vi "Set Message Type.vi"(6 "EF20 Message type":T1 items=["Update", "Graph", "Status", "Parameter", "Acknowledge"], 8 "error in":errorcluster, 11 "EF20 in":refnum<class "EF20.lvclass">) -> (0 "error out":errorcluster, 3 "EF20 out":refnum<class "EF20.lvclass">)   [LabVIEW 2018, in "EF20.lvlib" / "EF20.lvclass"]
uses:
  EF20.lvclass
  Custom Controls/EF20 Message Type.ctl
  EF20.lvclass/EF20.ctl
  EF20.lvlib
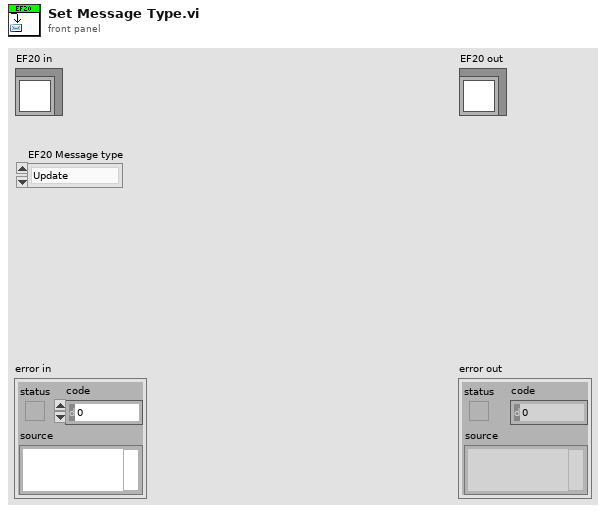
[diagram p1: front panel]
types:
  T1 = typedef "EF20.lvlib/EF20 Message Type.ctl" = u8
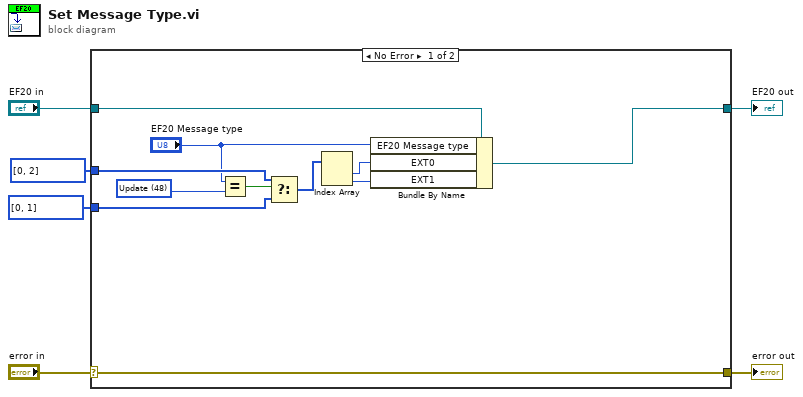
[diagram p0: block diagram]
diagram:
  n1 = case shown="No Error" "error in" {
    selector: "error in" -> [w17 w19]
    tunnel: [w17 w19] -> w5
    tunnel: [w15 w18] -> w3
    tunnel: "EF20 in" -> [w16 w18]
    tunnel: u8[] [0, 2] -> [w13 _]
    tunnel: u8[] [0, 1] -> [w12 _]
    frame No Error {
      w7 = T1 48 items=["Update"=48, "Graph"=49, "Status"=50, "Parameter"=51, "Acknowledge"=1] ("EF20 Message type")
      n2 = Equal?(x="EF20 Message type", y=w7) -> (x = y?=w14:bool)
      n3 = Select(t=w13, s=w14, f=w12) -> (s? t:f=w11:u8[])
      n4 = Index Array(array=w11) -> (element #1=w9:u8, element #2=w10:u8)  [unwired: 2 in]
      n5 = Bundle By Name(cluster=w16, "EF20 Message type"="EF20 Message type", "EXT0"=w9, "EXT1"=w10) -> (w15:refnum<class "EF20.lvclass">)
    }
    frame Error {
    }
  }
  "error out" <- w5
  "EF20 out" <- w3
